vi "Do.vi"(8 "error in (no error)":errorcluster, 10 "Actor in":refnum<class "Actor.lvclass">, 11 "Set Length Msg":refnum<class "Set Length Msg.lvclass">) -> (0 "error out":errorcluster, 2 "Actor out":refnum<class "Actor.lvclass">)   [LabVIEW 2020, in "BNT_ULx.lvlib" / "Set Length Msg.lvclass"]
doc: "This VI delivers the message to the actor by calling the appropriate method(s) on the actor."
uses:
  Set Length Msg.lvclass
  <vilib>/ActorFramework/Actor/Actor.lvclass
  C:/User/Brand/LVP/CSPP/CSPP-Template/Packages/CSPP_Core/Messages/CSPP_PVUpdate Msg/CSPP_PVUpdate Msg.lvclass
  CSPP_Core/Messages/CSPP_PVUpdate Msg/CSPP_PVUpdate Msg.lvclass/CSPP_PVUpdate Msg.ctl
  CSPP_Core/Classes/CSPP_ProcessVariables/ProcessVariable/PV.lvclass/PV.ctl
  Set Length Msg.lvclass/Set Length Msg.ctl
  CSPP_Core/Classes/CSPP_ProcessVariables/ProcessVariable/PV.lvclass
  <vilib>/regexp/Match Regular Expression.xnode
  CSPP_Core/Messages/CSPP_PVUpdate Msg/CSPP_PVUpdate Msg.lvclass
  BNT_ULx-MCSV-DOPWM/BNT_ULx-MCSV-DOPWM.lvclass
  C:/User/Brand/LVP/CSPP/CSPP-Template/Packages/CSPP_Core/Messages/CSPP_AsyncCallbackMsg/CSPP_AsyncCallback Msg.lvclass
  C:/Program Files (x86)/National Instruments/LabVIEW 2020/vi.lib/ActorFramework/Message/Message.lvclass
  C:/User/Brand/LVP/CSPP/CSPP-Template/Packages/BNT_ULx/BNT_ULx-MCSV/BNT_ULx-MCSV-DOPWM Messages/Set Length Msg/Set Length Msg.lvclass
  C:/User/Brand/LVP/CSPP/CSPP-Template/Packages/BNT_ULx/BNT_ULx-MCSV/BNT_ULx-MCSV/BNT_ULx-MCSV.lvclass
  C:/User/Brand/LVP/CSPP/CSPP-Template/Packages/CSPP_Core/Actors/CSPP_DeviceActor/CSPP_DeviceActor.lvclass
  C:/User/Brand/LVP/CSPP/CSPP-Template/Packages/CSPP_Core/Actors/CSPP_BaseActor/CSPP_BaseActor.lvclass
  C:/Program Files (x86)/National Instruments/LabVIEW 2020/vi.lib/ActorFramework/Actor/Actor.lvclass
  C:/User/Brand/LVP/CSPP/CSPP-Template/Packages/BNT_ULx/BNT_ULx-MCSV/BNT_ULx-MCSV-DOPWM/BNT_ULx-MCSV-DOPWM.lvclass
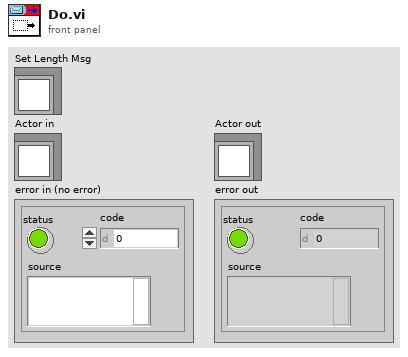
[diagram p1: front panel]
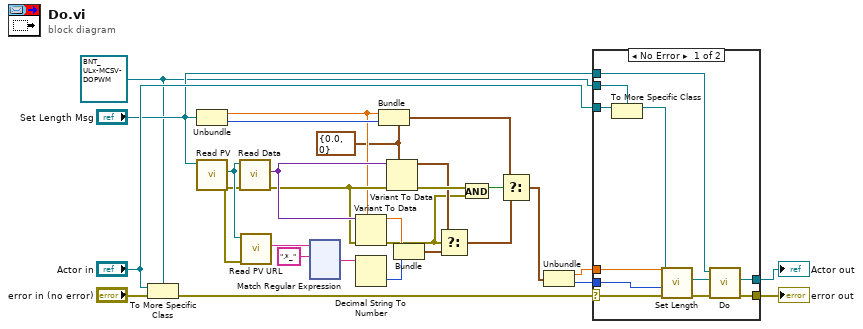
[diagram p0: block diagram]
diagram:
  w1 = refnum<class "BNT_ULx-MCSV-DOPWM.lvclass"> refnum ("BNT_ULx.lvlib:BNT_ULx-MCSV-DOPWM.lvclass")
  w2 = cluster{"PWM Length":dbl[unit], "Line":i32} {"PWM Length"=0.0, "Line"=0} ("cluster")
  n1 = To More Specific Class(target class=w1, reference="Actor in", error in="error in (no error)") -> (error out=w25:errorcluster)  [unwired: 1 out]
  n2 = Unbundle ("Pre-Unbundler")("Set Length Msg") -> (w10:dbl[unit], w20:i32)
  n3 = call "Read PV.vi"("CS++PVUpdate Msg in"="Set Length Msg") -> ("error out"=w13:errorcluster, "PV"=w14:refnum<class "PV.lvclass">)  [unwired: 8 in, 1 out]
  n4 = call "Read Data.vi"("error in (no error)"=w13, "PV in"=w14) -> ("error out"=w11:errorcluster, "Data"=w12:variant)  [unwired: 7 in, 1 out]
  n5 = call "Read PV URL.vi"("error in (no error)"=w13, "PV in"=w14) -> ("PV URL"=w19:string)  [unwired: 7 in, 2 out]
  n6 = xnode "Match Regular Expression"("input string"=w19, "regular expression"=".*_") -> ("after match"=w17:string)  [unwired: 4 in, 4 out]
  n7 = Variant To Data(error in=w11, type=w10, Variant=w12) -> (data=w9:dbl[unit], error out=w5:errorcluster)
  n8 = Decimal String To Number(string=w17) -> (number=w16:i32)  [unwired: 2 in, 1 out]
  n9 = Bundle ("Pre-Bundler")(cluster=w2, "PWM Length"=w10, "Line"=w20) -> (w21:cluster{"PWM Length":dbl[unit], "Line":i32})
  n10 = Variant To Data(error in=w11, type=w2, Variant=w12) -> (data=w8:cluster{"PWM Length":dbl[unit], "Line":i32}, error out=w22:errorcluster)
  n11 = Bundle ("Pre-Bundler")("PWM Length"=w9, w16) -> (w15:cluster{"PWM Length":dbl[unit], i32})  [unwired: 1 in]
  n12 = Select ("MainSelect")(t=w8, s=w5, f=w15) -> (s? t:f=w7:cluster{"PWM Length":dbl[unit], "Line":i32})
  n13 = And(x=w22, y=w5) -> (x .and. y?=w6:bool)
  n14 = Select ("MainSelect")(t=w21, s=w6, f=w7) -> (s? t:f=w4:cluster{"PWM Length":dbl[unit], "Line":i32})
  n15 = Unbundle ("Main-Unbundler")(w4) -> ("PWM Length"=w24:dbl[unit], "Line"=w23:i32)
  n16 = case shown="No Error" w25 {
    selector: w25 -> [w33 w42]
    tunnel: [w37 w42] -> w28
    tunnel: [w38 w41] -> w27
    tunnel: "Actor in" -> [w40 w41]
    tunnel: w1 -> [w39 _]
    tunnel: "Set Length Msg" -> [w36 _]
    tunnel: w24 -> [w35 _]
    tunnel: w23 -> [w34 _]
    frame No Error {
      n17 = To More Specific Class ("To More Specific Class (internal)")(target class=w39, reference=w40) -> (specific class reference=w32:refnum<class "BNT_ULx-MCSV-DOPWM.lvclass">)  [unwired: 1 in, 1 out]
      n18 = call "Set Length.vi"("error in"=w33, "Line"=w34, "PWM Length"=w35, "BNT_ULx-MCSV-DOPWM in"=w32) -> ("error out"=w30:errorcluster, "BNT_ULx-MCSV-DOPWM out"=w31:refnum<class "BNT_ULx-MCSV-DOPWM.lvclass">)  [unwired: 6 in]
      n19 = call-parent "Do.vi"("error in (no error)"=w30, "Actor in"=w31, "CS++PVUpdate Msg"=w36) -> ("error out"=w37:errorcluster, "Actor out"=w38:refnum<class "Actor.lvclass">)  [unwired: 7 in]
    }
    frame Error {
    }
  }
  "error out" <- w28
  "Actor out" <- w27
